vi "data buffer to string.vi"(1 "output pattern":digitaldata) -> (0 "initial string":string)   [LabVIEW 2012]
uses:
  <vilib>/Waveform/DWDTOps.llb/DWDT Digital to Binary U8.vi
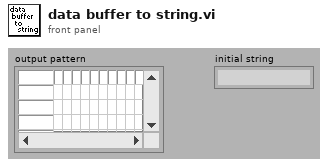
[diagram p1: front panel]
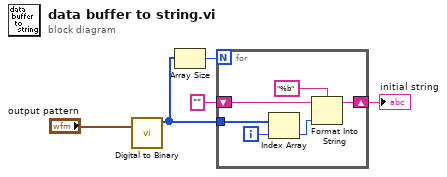
[diagram p0: block diagram]
diagram:
  n1 = call-poly <vilib>:"Digital to Binary.vi"("digital waveform"="output pattern") -> ("binary array"=w3:u8[])  [unwired: 1 in, 9 out]
  n2 = Array Size(array=w3) -> (size(s)=w2:i32)
  n3 = for {
    N: w2 -> [_]
    tunnel: w3 -> [w9]
    shift-right: [w8] -> w5
    shift-left: "" ("initial string") -> [w7]
    i -> [w10]
    n4 = Index Array(array=w9, index=w10) -> (element=w6:u8)
    n5 = Format Into String(format string="%b", initial string=w7, w6) -> (resulting string=w8:string)  [unwired: 1 in, 1 out]
  }
  "initial string" <- w5
